vi "Subpanel.vi"(5 "Panel Transparent":bool, 7 "Wait Until Done":bool, 8 "error in":errorcluster, 10 "Vi":path=path "C:/CT/Software/Panel/Configuration/GeneralConfigurationView.vi", 11 "SubPanel":refnum<vi>) -> (0 "error out":errorcluster, 2 "NextScreen":T1=enum."Config", 3 "ControlValues":cluster{"Name":string, "Variant Data":variant}[](array[cluster]))   [LabVIEW 2019]
uses:
  Telas.ctl
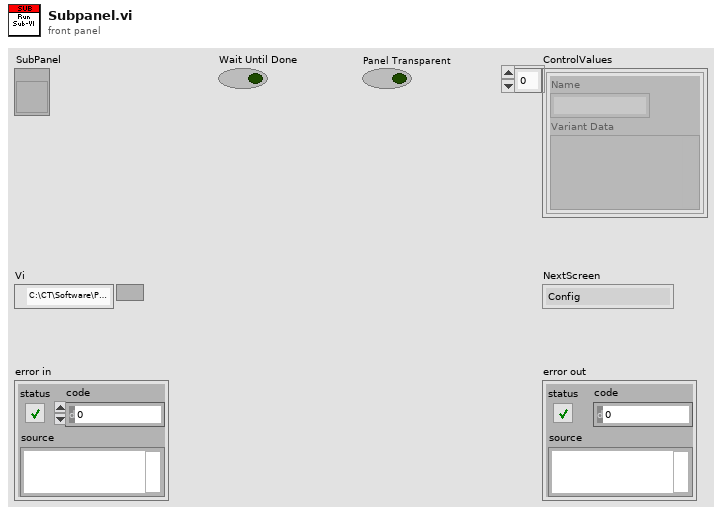
[diagram p1: front panel]
types:
  T1 = typedef "Telas.ctl" = enum16{"Selecao", "Config", "Medicao", "ParametrosTeste"}
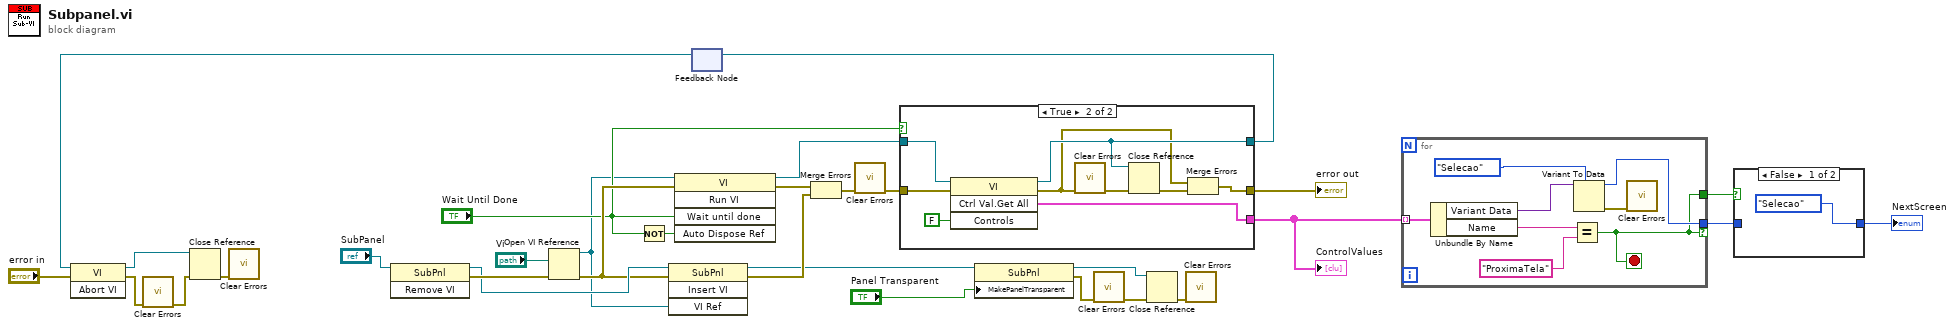
[diagram p0: block diagram]
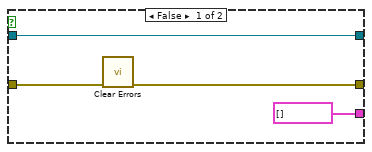
[diagram p2: hidden frame]
diagram:
  n1 = invoke on="Invoke Node" class="SubPnl" method="Remove VI"(reference="SubPanel") -> (reference out=w29:refnum<vi>, error out=w30:errorcluster)  [unwired: 2 in, 1 out]
  n2 = Open VI Reference(vi path="Vi", error in (no error)=w30) -> (vi reference=w7:refnum<vi>, error out=w11:errorcluster)  [unwired: 4 in]
  n3 = Not(x="Wait Until Done") -> (.not. x?=w16:bool)
  n4 = invoke on="Invoke Node" class="SubPnl" method="Insert VI"(reference=w29, error in=w11, "VI Ref"=w7) -> (reference out=w18:refnum<vi>, error out=w24:errorcluster)  [unwired: 1 in, 2 out]
  n5 = invoke class="VI" method="Run VI"(reference=w7, error in=w11, "Wait until done"="Wait Until Done", "Auto Dispose Ref"=w16) -> (reference out=w21:refnum<vi>, error out=w23:errorcluster)  [unwired: 1 in, 3 out]
  n6 = feedback #1() -> (w27:refnum<vi>)  [unwired: 1 in]
  n7 = invoke class="VI" method="Abort VI"(reference=w27, error in="error in") -> (reference out=w26:refnum<vi>, error out=w6:errorcluster)  [unwired: 1 in, 1 out]
  n8 = call <vilib>:"Clear Errors.vi"("error in (no error)"=w6) -> ("error out"=w5:errorcluster)  [unwired: 5 in, 1 out]
  n9 = Close Reference(reference=w26, error in (no error)=w5) -> (error out=w28:errorcluster)
  n10 = call <vilib>:"Clear Errors.vi"("error in (no error)"=w28) -> ()  [unwired: 5 in, 2 out]
  n11 = Merge Errors(w23, w24) -> (w22:errorcluster)
  n12 = call <vilib>:"Clear Errors.vi"("error in (no error)"=w22) -> ("error out"=w8:errorcluster)  [unwired: 5 in, 1 out]
  n13 = case shown="True" "Wait Until Done" {
    tunnel: w8 -> [w35 w41]
    tunnel: [w34 w38] -> w9
    tunnel: w21 -> [w33 w43]
    tunnel: [w33 w39] -> w20
    tunnel: [cluster{"Name":string, "Variant Data":variant}[] [] ("Get All Control Values Variant") w42] -> w15
    frame False {
      n14 = call <vilib>:"Clear Errors.vi"("error in (no error)"=w35) -> ("error out"=w34:errorcluster)  [unwired: 5 in, 1 out]
    }
    frame True {
      n15 = invoke class="VI" method="Ctrl Val.Get All"(reference=w43, error in=w41, "Controls"=FALSE) -> (reference out=w39:refnum<vi>, error out=w36:errorcluster, "Get All Control Values Variant"=w42:cluster{"Name":string, "Variant Data":variant}[])  [unwired: 1 in, 1 out]
      n16 = call <vilib>:"Clear Errors.vi"("error in (no error)"=w36) -> ("error out"=w37:errorcluster)  [unwired: 5 in, 1 out]
      n17 = Close Reference(reference=w39, error in (no error)=w37) -> (error out=w40:errorcluster)
      n18 = Merge Errors(w36, w40) -> (w38:errorcluster)
    }
  }
  "error out" <- w9
  "ControlValues" <- w15
  n19 = feedback-in #1(w20) -> ()
  n20 = property class="SubPnl"(reference=w18, "MakePanelTransparent"="Panel Transparent") -> (reference out=w1:refnum<vi>, error out=w2:errorcluster)  [unwired: 1 in]
  n21 = call <vilib>:"Clear Errors.vi"("error in (no error)"=w2) -> ("error out"=w4:errorcluster)  [unwired: 5 in, 1 out]
  n22 = Close Reference(reference=w1, error in (no error)=w4) -> (error out=w3:errorcluster)
  n23 = call <vilib>:"Clear Errors.vi"("error in (no error)"=w3) -> ()  [unwired: 5 in, 2 out]
  n24 = for {
    tunnel: w15 -> [w52] mode=indexing
    tunnel: [w49] -> w13 if=w48
    tunnel: [w48] -> w14
    stop <- w48 stop-if-true
    n25 = Unbundle By Name(w52) -> ("Variant Data"=w46:variant, "Name"=w47:string)
    n26 = Equal?(x=w47, y="ProximaTela") -> (x = y?=w48:bool)
    n27 = Variant To Data(type=Telas."Selecao" ("NextScreen"), Variant=w46) -> (data=w49:T1, error out=w50:errorcluster)  [unwired: 1 in]
    n28 = call <vilib>:"Clear Errors.vi"("error in (no error)"=w50) -> ()  [unwired: 5 in, 2 out]
  }
  n29 = case shown="False" w14 {
    tunnel: w13 -> [_ w54]
    tunnel: [Telas."Selecao" ("NextScreen") w54] -> w12
    frame False {
    }
    frame True {
    }
  }
  "NextScreen" <- w12
